vi "Create Measurement Service.vi"(8 "error in":errorcluster, 9 "measurement plug-in description":string, 10 "measurement plug-in name":string, 11 "project ref":refnum<vi>) -> (0 "error out":errorcluster)   [LabVIEW 2021, in "MeasurementService Editor.lvlib"]
uses:
  _MeasurementService Utility/MeasurementService Editor.lvlib
  _Generator Helpers/Generator Helpers.lvlib
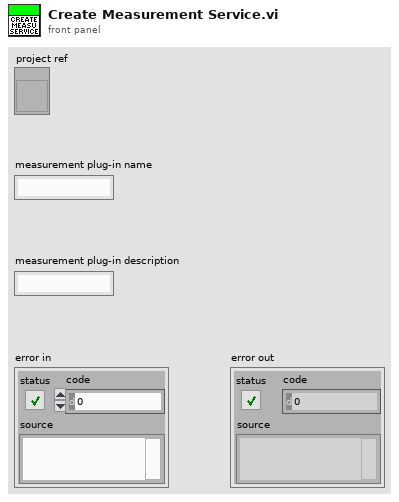
[diagram p1: front panel]
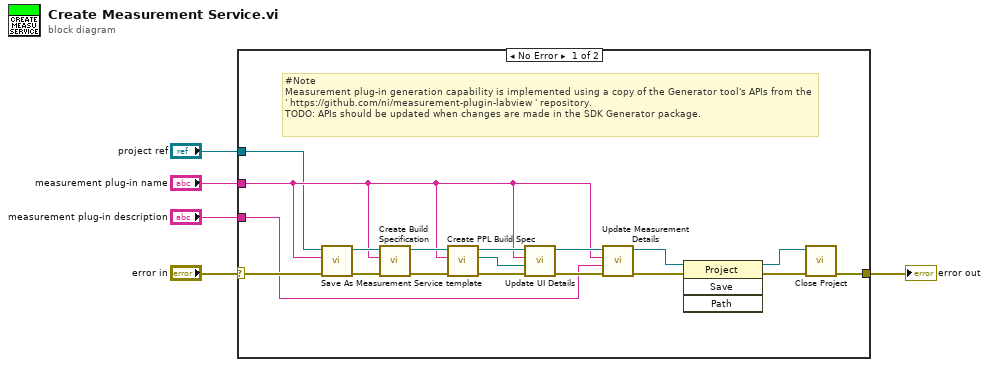
[diagram p0: block diagram]
diagram:
  n1 = case shown="No Error" "error in" {
    selector: "error in" -> [w13 w24]
    tunnel: [w8 w24] -> w1
    tunnel: "measurement plug-in name" -> [w12 _]
    tunnel: "project ref" -> [w7 _]
    tunnel: "measurement plug-in description" -> [w11 _]
    frame No Error {
      # "#Note\nMeasurement plug-in generation capability is implemented using a copy of the Generator tool's APIs from the ' https://github.com/ni/measurement-plugin-labview ' repository.\nTODO: APIs should be updated when changes are made in the SDK Generator package."
      n2 = call "Save As Measurement Service template.vi"("error in"=w13, "measurement service name"=w12, "project ref"=w7) -> ("error out"=w19:errorcluster, "project ref out"=w18:refnum<vi>)  [unwired: 7 in]
      n3 = call "Create Build Specification.vi"("error in"=w19, "measurement service name"=w12, "project ref"=w18) -> ("error out"=w22:errorcluster, "project ref out"=w17:refnum<vi>)  [unwired: 7 in]
      n4 = call "Create PPL Build Spec.vi"("error in (no error)"=w22, "measurement plug-in name"=w12, "project refnum"=w17) -> ("error out"=w21:errorcluster, "measurement UI built path"=w6:path, "project ref out"=w16:refnum<vi>)  [unwired: 6 in]
      n5 = call "Update UI Details.vi"("error in"=w21, "UI path"=w6, "measurement service name"=w12, "project ref"=w16) -> ("error out"=w20:errorcluster, "project ref out"=w15:refnum<vi>)  [unwired: 6 in]
      n6 = call "Update Measurement Details.vi"("error in"=w20, "measurement service description"=w11, "measurement service name"=w12, "project ref"=w15) -> ("error out"=w23:errorcluster, "project ref out"=w10:refnum<vi>)  [unwired: 6 in]
      n7 = invoke class="Project" method="Save"(reference=w10, error in=w23) -> (reference out=w9:refnum<vi>, error out=w14:errorcluster)  [unwired: 2 in, 2 out]
      n8 = call "Close Project.vi"("error in"=w14, "project ref"=w9) -> ("error out"=w8:errorcluster)  [unwired: 9 in]
    }
    frame Error {
    }
  }
  "error out" <- w1
